vi "Configure Setpoints Limits.vi"(0 "VISA resource name":refnum<visa-resource-name>, 1 "Unit Address (1)":u8=1 min=1 max=254, 5 "Setpoint Limit (0:Low)":u16(ring) items=["Low", "High"], 9 "Setpoint Limit Value (0)":sgl, 11 "error in (no error)":errorcluster) -> (4 "VISA resource name out":refnum<visa-resource-name>, 15 "error out":errorcluster)   [LabVIEW 2010, in "Eurotherm 32xx Series.lvlib"]
doc: "This VI sets Setpoints limits."
uses:
  <instrlib>/Eurotherm 32xx Series/Eurotherm 32xx Series.lvlib
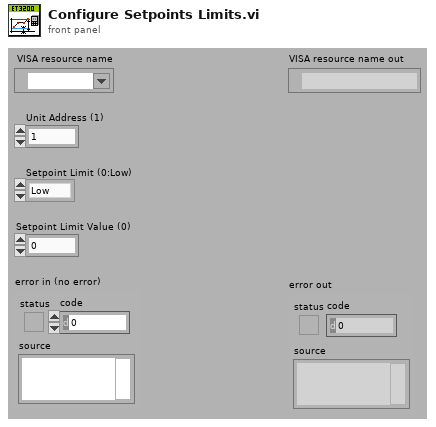
[diagram p1: front panel]
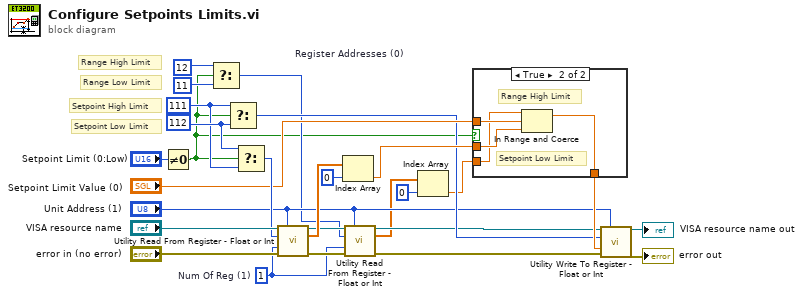
[diagram p0: block diagram]
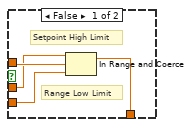
[diagram p2: hidden frame]
diagram:
  w4 = u16 1  # Num Of Reg (1)
  w23 = u16 112 ("Register Addresses (0)")
  w22 = u16 111  # Register Addresses (0)
  # "Setpoint Low Limit"
  # "Setpoint High Limit"
  # "Range Low Limit"
  # "Range High Limit"
  n1 = Not Equal To 0?(x="Setpoint Limit (0:Low)") -> (x != 0?=w1:bool)
  n2 = Select(t=u16 12 ("Register Addresses (0)"), s=w1, f=u16 11 ("Register Addresses (0)")) -> (s? t:f=w5:u16)
  n3 = Select(t=w22, s=w1, f=w23) -> (s? t:f=w15:u16)
  n4 = Select(t=w23, s=w1, f=w22) -> (s? t:f=w21:u16)
  n5 = call <instrlib>:"Utility Read From Register - Float or Int.vi"("VISA resource name"="VISA resource name", "Unit Address (1)"="Unit Address (1)", "Register Address (0)"=w21, "Num Of Reg (1)"=w4, "error in (no error)"="error in (no error)") -> ("VISA resource name out"=w11:refnum<visa-resource-name>, "Data"=w20:sgl[], "error out"=w14:errorcluster)  [unwired: 8 in]
  n6 = Index Array(array=w20, index=0) -> (element=w18:sgl)
  n7 = call <instrlib>:"Utility Read From Register - Float or Int.vi"("VISA resource name"=w11, "Unit Address (1)"="Unit Address (1)", "Register Address (0)"=w5, "Num Of Reg (1)"=w4, "error in (no error)"=w14) -> ("VISA resource name out"=w12:refnum<visa-resource-name>, "Data"=w8:sgl[], "error out"=w13:errorcluster)  [unwired: 8 in]
  n8 = Index Array(array=w8, index=0) -> (element=w3:sgl)
  n9 = case shown="True" w1 {
    tunnel: w18 -> [w30 w35]
    tunnel: "Setpoint Limit Value (0)" -> [w31 w34]
    tunnel: [w29 w33] -> w16
    tunnel: w3 -> [w28 w32]
    frame False {
      # "Range Low Limit"
      # "Setpoint High Limit"
      n10 = In Range and Coerce(upper limit=w30, x=w31, lower limit=w28) -> (coerced(x)=w29:sgl)  [unwired: 1 out]
    }
    frame True {
      # "Range High Limit"
      # "Setpoint Low Limit"
      n11 = In Range and Coerce(upper limit=w32, x=w34, lower limit=w35) -> (coerced(x)=w33:sgl)  [unwired: 1 out]
    }
  }
  n12 = call <instrlib>:"Utility Write To Register - Float or Int.vi"("VISA resource name"=w12, "Unit Address (1)"="Unit Address (1)", "Register Address (0)"=w15, "Data (0)"=w16, "error in (no error)"=w13) -> ("VISA resource name out"=→"VISA resource name out":refnum<visa-resource-name>, "error out"=→"error out":errorcluster)  [unwired: 9 in]
